vi "SineWaveIdent.vi"() -> ()   [LabVIEW 2015]
uses:
  <vilib>/Platform/TimedLoop/XDataNode/timing_clust.ctl
  <vilib>/Platform/TimedLoop/XDataNode/nitl_modes.ctl
  <vilib>/Platform/TimedLoop/XDataNode/wakeup.ctl
  <vilib>/FPGAPlugInAG/myRIO-1900/niLvFpga_Open_myRIO-1900.vi
  <vilib>/rvi/interface/common/dynamic/niFpgaDynamicAddResources.vi
  <vilib>/Utility/file.llb/Write Delimited Spreadsheet (DBL).vi
  <vilib>/Utility/error.llb/Error Cluster From Error Code.vi
  <vilib>/rvi/errors/niLvFpgaAdjustHostInterfaceError.vi
  <vilib>/FPGAPlugInAG/Dynamic/niLvFpga_Close_Dynamic.vi
  <vilib>/rvi/interface/nirviOpenFPGA/nirviOpenFPGA.xnode
  FPGA Bitfiles/ViconProj_FPGATarget_CurrentControlle_KJVtLDFLiQk.lvbitx
  Misc/Current Controller.vi
  <vilib>/Platform/TimedLoop/XDataNode/XDataNode.xnode
  <vilib>/rvi/interface/nirviReadWriteControl/nirviReadWriteControl.xnode
  <vilib>/rvi/interface/nirviCloseFPGA/nirviCloseFPGA.xnode
  <vilib>/rvi/interface/Simulation/niFpgaSimulationCallBeginRW.vi
  <vilib>/Platform/TimedLoop/XDataNode/XDNodeRunTimeDep.lvlib
  NiFpgaLv.dll
  <vilib>/Analysis/NI_AALBase.lvlib
  <vilib>/ptbypt/NI_PtbyPt.lvlib
panel:
  in  "Spectral Amplitude":dbl(knob)=16.254291221099862 scale=60.0..170.0
  out "Pose":dbl[][](array[numeric])
  in  "Tab Control 2":enum32{"Page 1"}(tab)
  in  "Stop":bool
  in  "Tab Control":enum32{"Monitor", "Monitor 2"}(tab)
  out "Sine Val":dbl
  out "Sine Wave":dbl[](graph)
  out "FPGA Status":bool
  out "yaw":dbl
  out "pitch":dbl
  out "roll":dbl
  out "y":dbl
  out "z":dbl
  out "x":dbl
  out "PoseVect":dbl[][](graph)
  in  "Amplitude":dbl(knob)=16.254291221099862 scale=60.0..170.0
  out "FPGA Loop error":errorcluster
  out "FPGA TImed Loop error":errorcluster
  out "UWGN Error":errorcluster
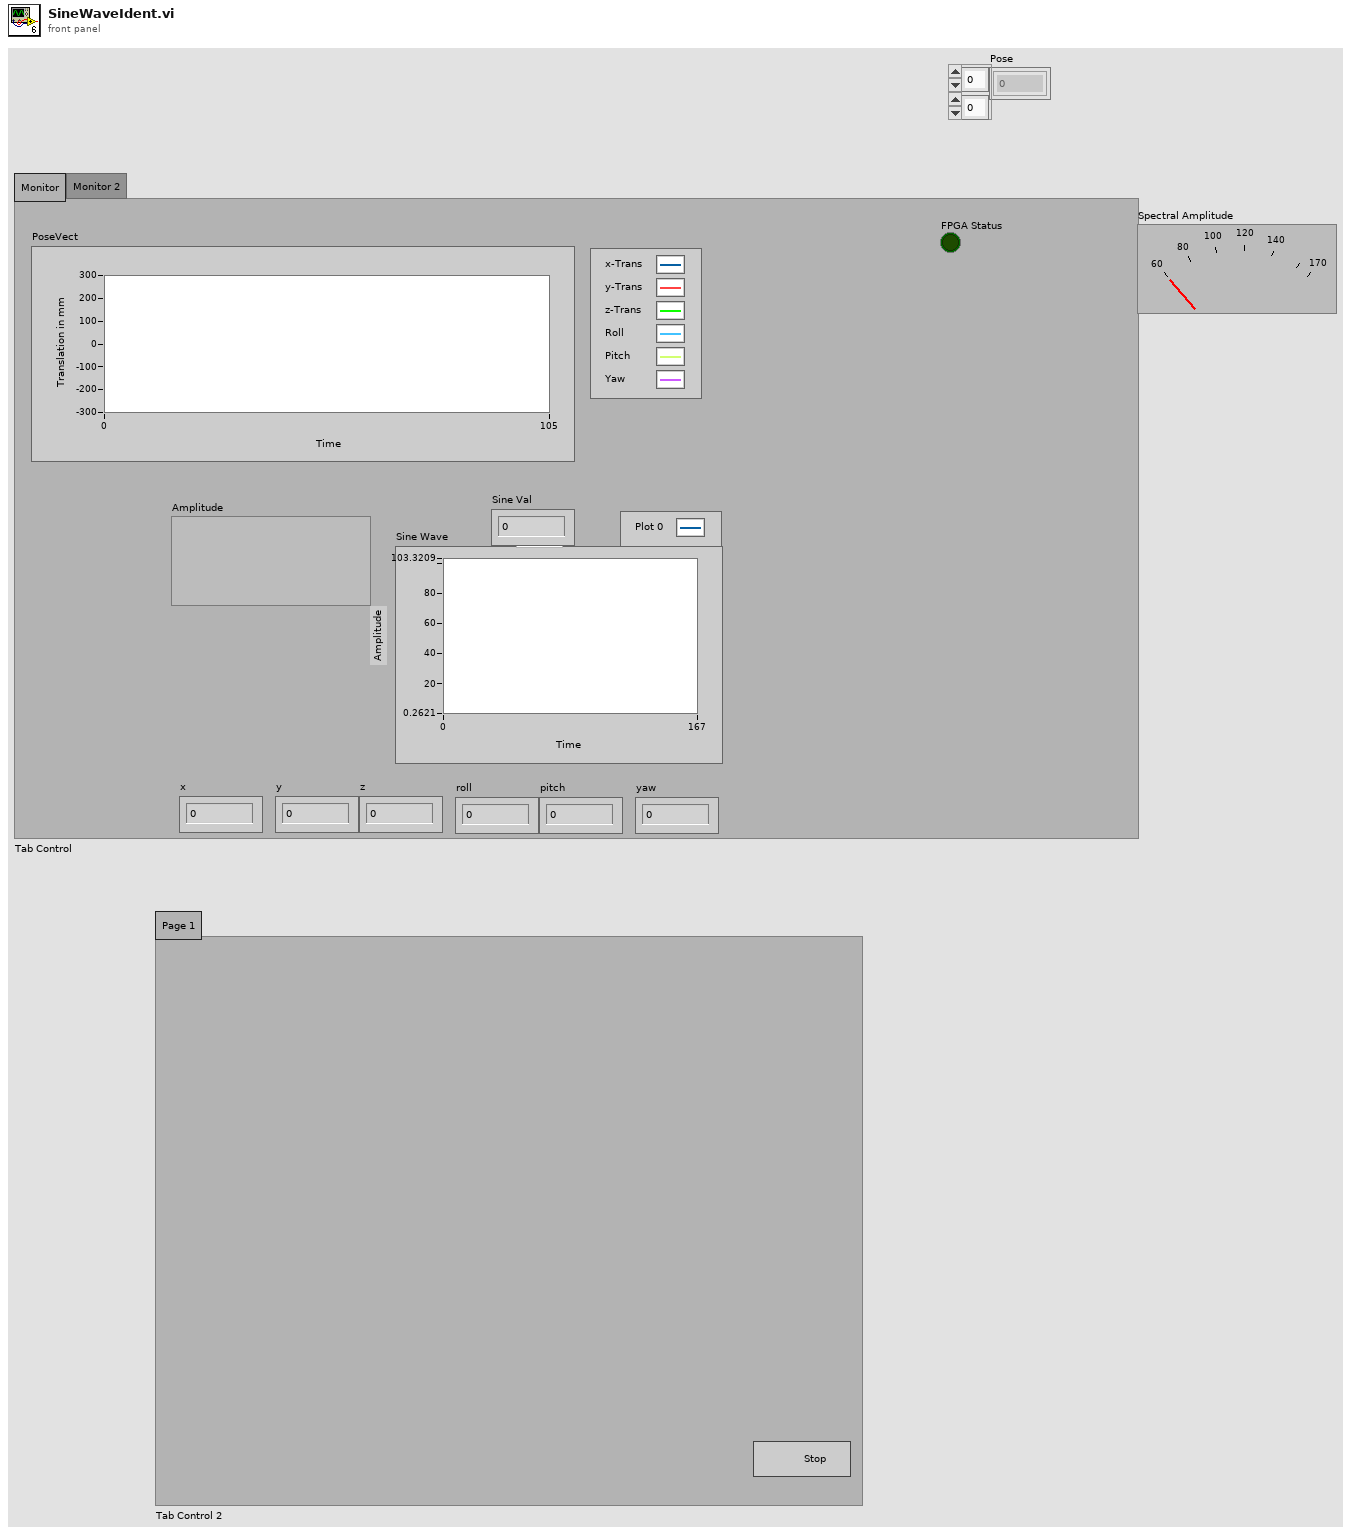
[diagram p1: front panel]
types:
  T1 = typedef "XDNodeRunTimeDep.lvlib/timing_clust.ctl" = cluster{"Expected End [f-1]":u64, "Actual End [f-1]":u64, "Finished Late? [f-1]":bool, "Expected End [i-1]":u64, "Actual End [i-1]":u64, "Finished Late? [i-1]":bool, "Expected Start [i]":u64, "Actual Start [i]":u64, "Expected Start [f]":u64, "Actual Start [f]":u64, "Source Name":string, "Structure Name":string, "Period":i64, "Deadline":i64, "Offset":i64, "Start":i64, "Priority":i32, "Timeout":i32, "Mode":T2, "Wakeup Reason":T3, "Error":errorcluster, "Source Type":string, "Secondary Source Type":string, "Global End Time":u64, "Global Start Time":u64, "Frame Duration":u64, "Iteration Duration":u64, "Assigned CPU":i32, "I/O Scan Engine Mode":u32}
  T2 = typedef "XDNodeRunTimeDep.lvlib/nitl_modes.ctl" = enum32{"No Change", "Process missed periods, maintain original phase", "Discard missed periods, maintain original phase", "Process missed periods, ignore original phase", "Discard missed periods, ignore original phase"}
  T3 = typedef "XDNodeRunTimeDep.lvlib/wakeup.ctl" = enum32{"Normal", "Aborted", "Asynchronous wakeup", "Timing source error", "Timed loop error", "Timeout"}
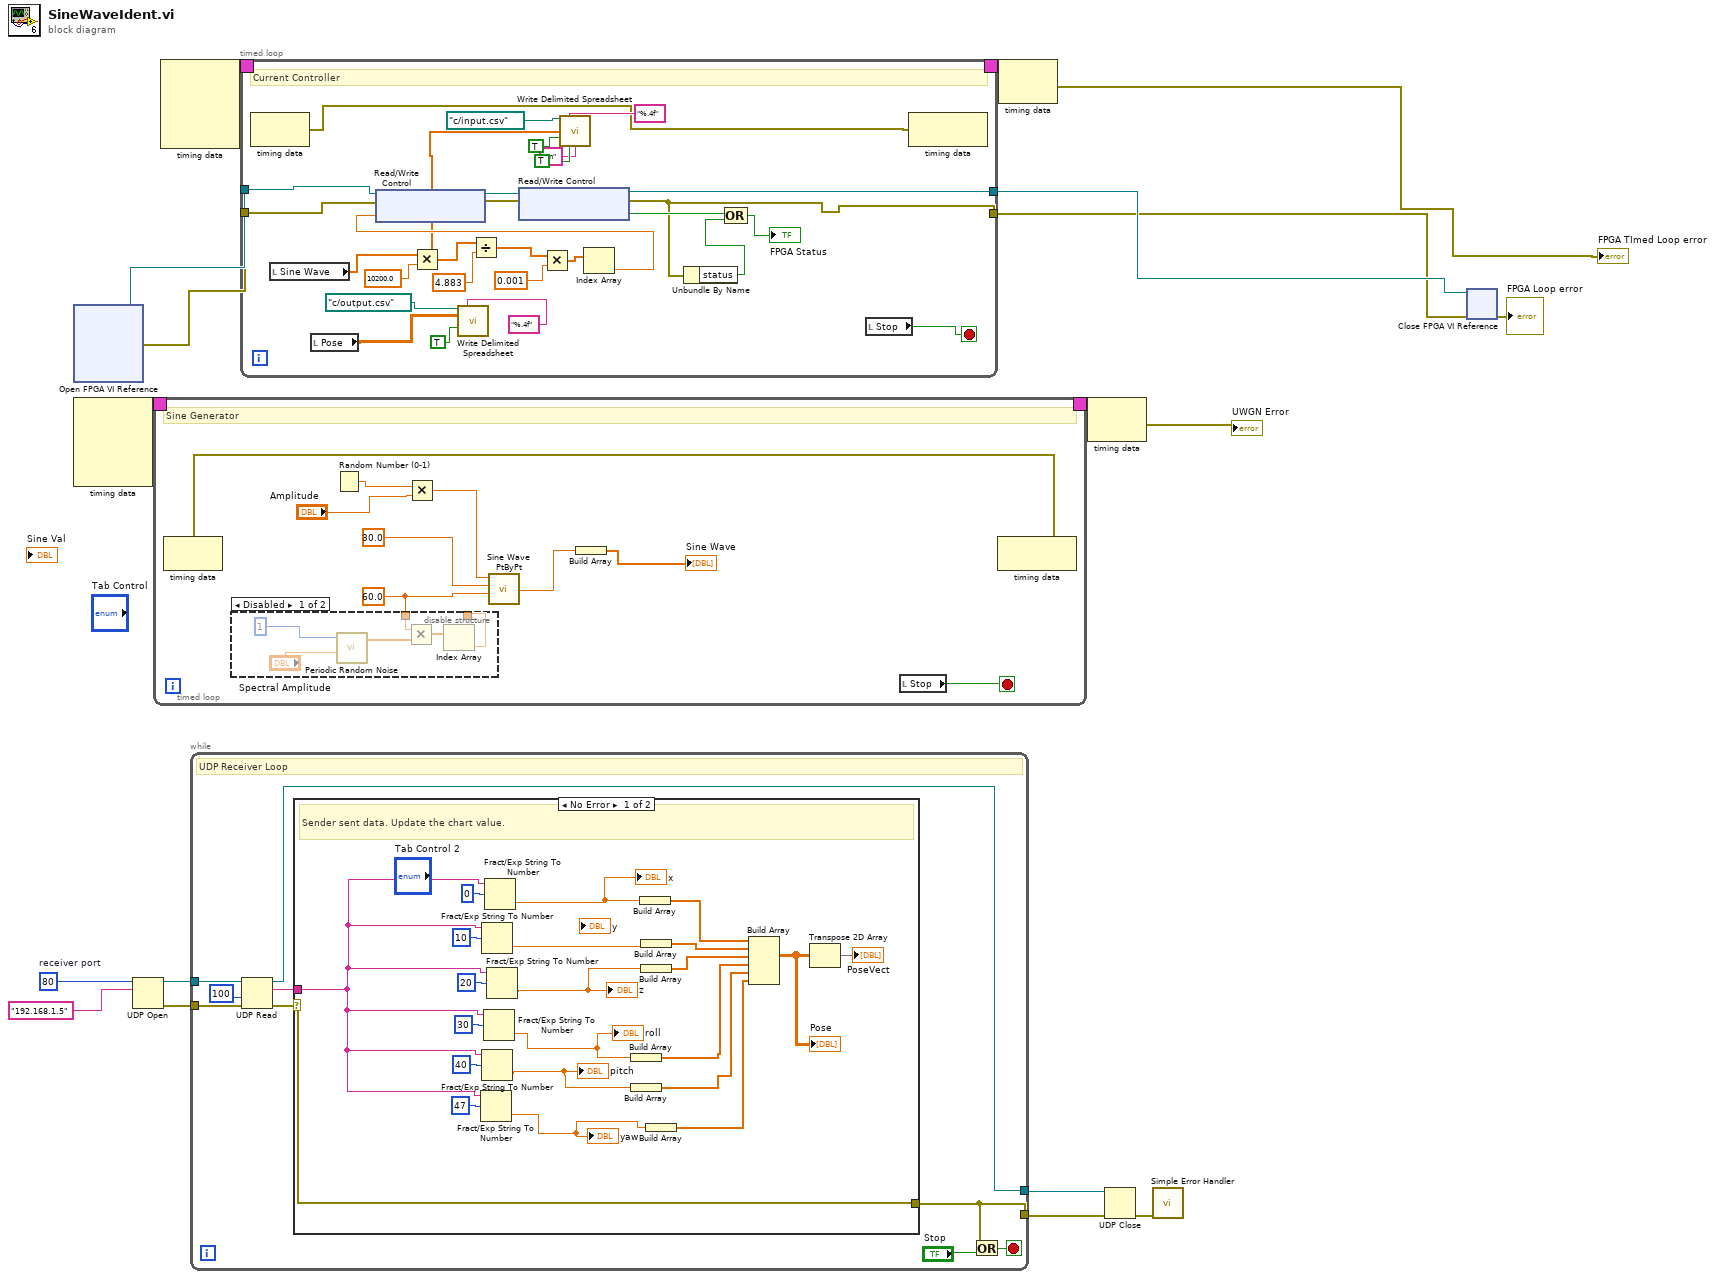
[diagram p0: block diagram]
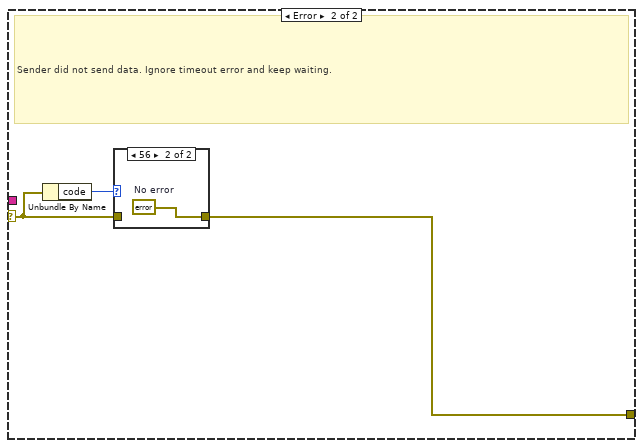
[diagram p2: hidden frame]
diagram:
  w2 = u16 80  # receiver port
  n1 = xnode "Open FPGA VI Reference"() -> ("FPGA VI Reference Out"=w18:refnum<k20>, "error out"=w17:errorcluster)  [unwired: 2 in]
  n2 = node-c288() -> (w14:T1)  [unwired: 4 in]
  n3 = UDP Open(10:"192.168.1.5" ("service name"), 11:w2) -> (port=w3:refnum<k16>, 0:w4:errorcluster)  [unwired: 3 in, 1 out]
  n4 = timed-loop {
    timing: w14 -> [_]
    timing-out: [_] -> w13
    stop <- w26 stop-if-true
    w22 = 60.0 ("phase(degrees)")
    # "Sine Generator"
    n5 = node-c288() -> (w27:errorcluster)  [unwired: 1 in]
    n6 = disable-structure shown="Disabled" {
      disable-tunnel: w22 -> [w33 _]
      disable-tunnel: [w28 _] -> _
      frame Disabled {
        n7 = call <vilib>:"Periodic Random Noise.vi"("spectral amplitude"="Spectral Amplitude", "samples"=1) -> ("periodic random noise"=w32:dbl[])  [unwired: 1 in, 1 out]
        n8 = Multiply(x=w33, y=w32) -> (x*y=w29:dbl[])
        n9 = Index Array(array=w29) -> (element=w28:dbl)  [unwired: 1 in]
      }
      frame Enabled {
      }
    }
    n10 = Random Number (0-1)() -> (number: 0 to 1=w20:dbl)
    n11 = Multiply(x=w20, y="Amplitude") -> (x*y=w19:dbl)
    n12 = call <vilib>:"Sine Wave PtByPt.vi"("phase"=w22, "frequency"=30.0, "amplitude"=w19) -> ("sine wave"=w24:dbl)  [unwired: 1 in]
    n13 = Build Array(w24) -> (→"Sine Wave":dbl[])
    n14 = local read "Stop"() -> (w26:bool)
    n15 = node-c288(w27) -> ()  [unwired: 1 out]
  }
  n16 = node-c288() -> (w12:T1)  [unwired: 4 in]
  n17 = while {
    tunnel: w3 -> [w47]
    tunnel: [w39] -> w7
    tunnel: w4 -> [w44]
    tunnel: [w40] -> w5
    stop <- w45 stop-if-true
    # "UDP Receiver Loop"
    n18 = UDP Read(connection ID=w47, timeout ms (25000)=100, 8:w44) -> (data out=w42:string, error out=w41:errorcluster, 3:w39:refnum<k16>)  [unwired: 3 out]
    n19 = case shown="No Error" w41 {
      selector: w41 -> [w69 w71]
      tunnel: w42 -> [w59 _]
      tunnel: [w69 w70] -> w40
      frame No Error {
        # "Sender sent data. Update the chart value."
        n20 = Fract/Exp String To Number(string=w59, offset=47) -> (number=w51:dbl)  [unwired: 2 in, 1 out]
        "yaw" <- w51
        n21 = Fract/Exp String To Number(string=w59, offset=10) -> (number=w49:dbl)  [unwired: 2 in, 1 out]
        n22 = Fract/Exp String To Number(string=w59, offset=40) -> (number=w52:dbl)  [unwired: 2 in, 1 out]
        "pitch" <- w52
        n23 = Fract/Exp String To Number(string=w59, offset=30) -> (number=w53:dbl)  [unwired: 2 in, 1 out]
        "roll" <- w53
        n24 = Fract/Exp String To Number(string=w59, offset=0) -> (number=w50:dbl)  [unwired: 2 in, 1 out]
        "x" <- w50
        n25 = Fract/Exp String To Number(string=w59, offset=20) -> (number=w48:dbl)  [unwired: 2 in, 1 out]
        "z" <- w48
        n26 = Build Array(w53) -> (w56:dbl[])
        n27 = Build Array(w52) -> (w55:dbl[])
        n28 = Build Array(w50) -> (w61:dbl[])
        n29 = Build Array(w49) -> (w60:dbl[])
        n30 = Build Array(w48) -> (w65:dbl[])
        n31 = Build Array(w51) -> (w54:dbl[])
        n32 = Build Array(w61, w60, w65, w56, w55, w54) -> (w58:dbl[][])
        "Pose" <- w58
        n33 = Transpose 2D Array(2D array=w58) -> (transposed array=→"PoseVect":dbl[][])
      }
      frame Error {
        # "Sender did not send data. Ignore timeout error and keep waiting."
        n34 = Unbundle By Name(w71) -> ("code"=w72:i32)
        n35 = case shown="56" w72 {
          tunnel: w71 -> [w73 _]
          tunnel: [w73 w74] -> w70
          frame Default {
          }
          frame 56 {
            w74 = errorcluster {"status"=FALSE, "code"=0, "source"=""}  # No error
          }
        }
      }
    }
    n36 = Or(x=w40, y="Stop") -> (x .or. y?=w45:bool)
  }
  n37 = timed-loop {
    tunnel: w18 -> [w102]
    tunnel: w17 -> [w101]
    tunnel: [w93] -> w16
    tunnel: [w90] -> w15
    timing: w12 -> [_]
    timing-out: [_] -> w11
    stop <- w77 stop-if-true
    # "Current Controller"
    n38 = node-c288() -> (w80:errorcluster)  [unwired: 1 in]
    n39 = local read "Sine Wave"() -> (w75:dbl[])
    n40 = local read "Pose"() -> (w76:dbl[][])
    n41 = Multiply(x=w75, y=10200.0) -> (x*y=w97:dbl[])
    n42 = call-poly <vilib>:"Write Delimited Spreadsheet.vi"("file path (dialog if empty)"=path "c:/output.csv", "format (%.3f)"="%.4f", "2D data"=w76, "append to file? (F)"=TRUE) -> ()  [unwired: 10 in, 2 out]
    n43 = Divide(x=w97, y=4.883) -> (x/y=w99:dbl[])
    n44 = Multiply(x=w99, y=0.001) -> (x*y=w82:dbl[])
    n45 = call-poly <vilib>:"Write Delimited Spreadsheet.vi"("file path (dialog if empty)"=path "c:/input.csv", "format (%.3f)"="%.4f" ("format (%d)"), "1D data"=w75, "append to file? (F)"=TRUE, "transpose? (F)"=TRUE, "delimiter (\\t)"="\\n" ("delimiter (\\t)")) -> ()  [unwired: 8 in, 2 out]
    n46 = Index Array(array=w82) -> (element=w81:dbl)  [unwired: 1 in]
    n47 = xnode "Read/Write Control"("FPGA VI Reference In"=w102, "error in"=w101, "DAC Outlet Valve"=w81) -> ("FPGA VI Reference Out"=w95:refnum<k20>, "error out"=w94:errorcluster)
    n48 = xnode "Read/Write Control"("FPGA VI Reference In"=w95, "error in"=w94) -> ("FPGA VI Reference Out"=w93:refnum<k20>, "error out"=w90:errorcluster, "Outlet Overflow?"=w91:bool)
    n49 = Unbundle By Name(w90) -> ("status"=w92:bool)
    n50 = Compound Arithmetic op=OR(w91, w92) -> (→"FPGA Status":bool)
    n51 = local read "Stop"() -> (w77:bool)
    n52 = node-c288(w80) -> ()  [unwired: 1 out]
  }
  n53 = node-c288(w11) -> (→"FPGA TImed Loop error":errorcluster)
  n54 = node-c288(w13) -> (→"UWGN Error":errorcluster)
  n55 = UDP Close(connection ID=w7, 8:w5) -> (error out=w6:errorcluster)  [unwired: 1 out]
  n56 = call <vilib>:"Simple Error Handler.vi"("error in (no error)"=w6) -> ()  [unwired: 1 in, 8 out]
  n57 = xnode "Close FPGA VI Reference"("FPGA VI Reference In"=w16, "error in"=w15) -> ("error out"=→"FPGA Loop error":errorcluster)
